vi "Pre Launch Init.vi"(11 "Iterator Actor in":refnum<class "Iterator NR Actor.lvclass">) -> (0 "error out":errorcluster, 3 "Iterator Actor out":refnum<class "Iterator NR Actor.lvclass">)   [LabVIEW 2023, in "Iterator Actor.lvlib" / "Iterator NR Actor.lvclass"]
doc: "(<B>Filename</B>: Actor Framework.lvlib:Actor.lvclass:Pre Launch Init.vi)\n\nDefines behavior that occurs after the Launch Nested Actor method is invoked but before the actor's Actor Core method begins running.\n\nBy default, this method does nothing. A descendant class may override it to define behavior."
uses:
  Iterator NR Actor.lvclass
  <vilib>/ActorFramework/Actor/Actor.lvclass/Actor.ctl
  <vilib>/ActorFramework/Message Enqueuer/Message Enqueuer.lvclass/Message Enqueuer.ctl
  Iterator NR Actor.lvclass/Iterator NR Actor.ctl
  Iterator NR Actor Messages/Request Iteration Notification Msg/Request Iteration Notification Msg.lvclass
  Iterator NR Actor Messages/Request Iteration Notification Msg/Request Iteration Notification Msg.lvclass/Request Iteration Notification Msg.ctl
  Iterator NR Actor Messages/Request Iteration Notification Msg/Write Iterator Enqueuer.vi
  <vilib>/ActorFramework/Message Enqueuer/Init from Existing Queue.vi
  Abstract Iterator Actor/Abstract Iterator Actor.lvclass
  <vilib>/ActorFramework/Message Enqueuer/Message Enqueuer.lvclass
  <userlib>/_OpenG.lib/error/error.llb/openg_error.lvlib
  <vilib>/ActorFramework/Actor/Actor.lvclass
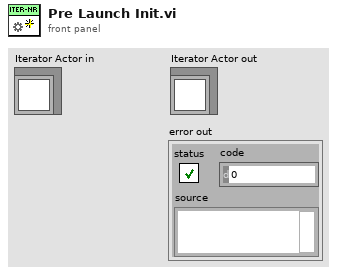
[diagram p1: front panel]
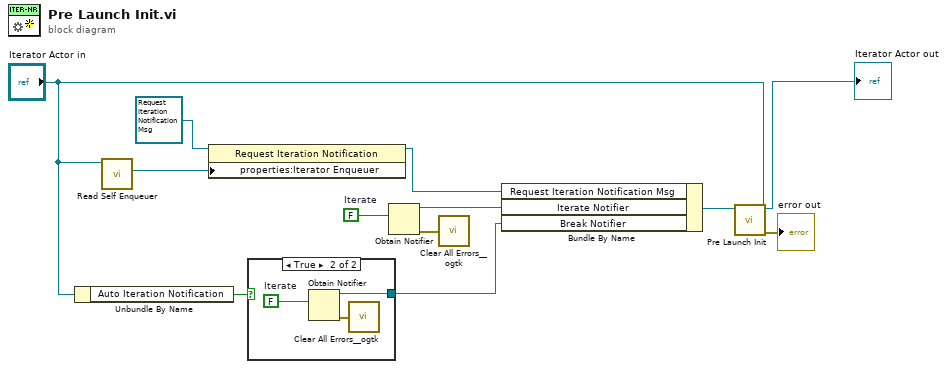
[diagram p0: block diagram]
diagram:
  w9 = FALSE  # Iterate
  n1 = Unbundle By Name("Iterator Actor in") -> ("Auto Iteration Notification"=w2:bool)
  n2 = call <vilib>:"Read Self Enqueuer.vi"("Actor"="Iterator Actor in") -> ("Self Enqueuer"=w4:refnum<class "Message Enqueuer.lvclass">)  [unwired: 10 in]
  n3 = property class="Request Iteration Notification "(reference=refnum<class "Request Iteration Notification Msg.lvclass"> refnum ("Iterator Actor.lvlib:Request Iteration Notification Msg.lvclass"), "properties:Iterator Enqueuer"=w4) -> (reference out=w5:refnum<class "Request Iteration Notification Msg.lvclass">)  [unwired: 1 in, 1 out]
  n4 = case shown="True" w2 {
    tunnel: [_ w13] -> w1
    frame False {
    }
    frame True {
      w15 = FALSE  # Iterate
      n5 = Obtain Notifier(notification data type=w15) -> (notifier out=w13:refnum<notifier>, error out=w14:errorcluster)  [unwired: 3 in, 1 out]
      n6 = call <userlib>:"Clear All Errors__ogtk.vi"("Error In"=w14) -> ()  [unwired: 3 in, 1 out]
    }
  }
  n7 = Obtain Notifier(notification data type=w9) -> (notifier out=w8:refnum<notifier>, error out=w7:errorcluster)  [unwired: 3 in, 1 out]
  n8 = call <userlib>:"Clear All Errors__ogtk.vi"("Error In"=w7) -> ()  [unwired: 3 in, 1 out]
  n9 = Bundle By Name(cluster="Iterator Actor in", "Request Iteration Notification Msg"=w5, "Iterate Notifier"=w8, "Break Notifier"=w1) -> (w10:refnum<class "Iterator NR Actor.lvclass">)
  n10 = call-parent "Pre Launch Init.vi"("Iterator Actor in"=w10) -> ("error out"=→"error out":errorcluster, "Iterator Actor out"=→"Iterator Actor out":refnum<class "Iterator NR Actor.lvclass">)  [unwired: 9 in]
